vi "Read Swiat Size.vi"(8 "error in (no error)":errorcluster, 11 "Swiat in":refnum<class "Swiat.lvclass">) -> (0 "error out":errorcluster, 2 "Size out":T1, 3 "Swiat out":refnum<class "Swiat.lvclass">)   [LabVIEW 2014, in "Swiat.lvclass"]
uses:
  Swiat.lvclass
  <vilib>/Utility/miscctls.llb/LVBoundsTypeDef.ctl
  Swiat.lvclass/Swiat.ctl
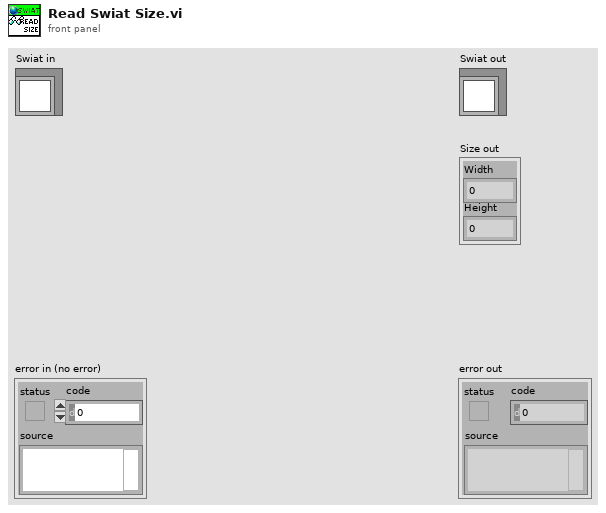
[diagram p1: front panel]
types:
  T1 = typedef "LVBoundsTypeDef.ctl" = cluster{"Width":u32, "Height":u32}
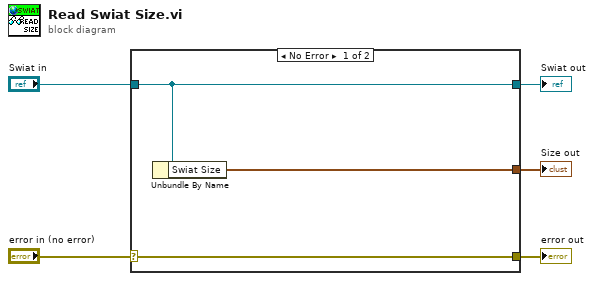
[diagram p0: block diagram]
diagram:
  n1 = case shown="No Error" "error in (no error)" {
    selector: "error in (no error)" -> [w8 w9]
    tunnel: [w8 w9] -> w4
    tunnel: [w7 w10] -> w2
    tunnel: "Swiat in" -> [w7 w10]
    tunnel: [w6 _] -> w1
    frame No Error {
      n2 = Unbundle By Name(w7) -> ("Swiat Size"=w6:T1)
    }
    frame Error {
    }
  }
  "error out" <- w4
  "Swiat out" <- w2
  "Size out" <- w1
